vi "MFLIcontrol.vi"(6 "SigIns0 Autorange":bool, 7 "Value":dbl, 8 "error in":errorcluster, 10 "MFLI function":T2, 11 "handle in":T3 {"Handle" format="0x%08x"; "Conn" format="0x%08x"}) -> (0 "error out":errorcluster, 1 "Demod Sample Out 2":T1={"Timestamps (ticks)"=0, "X (Vrms)"=nan, "Y (Vrms)"=nan, "Osc Phase (deg)"=nan, "Freq (Hz)"=nan, "DIO"=0, "AuxIn0 (V)"=nan, "AuxIn1 (V)"=nan, "Trigger"=0}, 2 "Demod Sample Out 3":T1={"Timestamps (ticks)"=0, "X (Vrms)"=nan, "Y (Vrms)"=nan, "Osc Phase (deg)"=nan, "Freq (Hz)"=nan, "DIO"=0, "AuxIn0 (V)"=nan, "AuxIn1 (V)"=nan, "Trigger"=0}, 3 "handle out":T3 {"Handle" format="0x%08x"; "Conn" format="0x%08x"}, 4 "AuxOut0_Ampl":dbl)   [LabVIEW 2021]
uses:
  <instrlib>/Zurich Instruments LabOne/Public/ziTypeHandle.ctl
  MFLIcommand.ctl
  <instrlib>/Zurich Instruments LabOne/Public/Data/ziTypeDemodSampleSingle.ctl
  <instrlib>/Zurich Instruments LabOne/Public/Configure/ziGetValueDemodSampleEx.vi
  <instrlib>/Zurich Instruments LabOne/Public/Configure/ziSetValueDouble.vi
  <instrlib>/Zurich Instruments LabOne/Public/Configure/ziGetValueDouble.vi
  <instrlib>/Zurich Instruments LabOne/Zurich Instruments LabOne.lvlib
panel:
  out "Demod Sample Out 5":T1={"Timestamps (ticks)"=0, "X (Vrms)"=nan, "Y (Vrms)"=nan, "Osc Phase (deg)"=nan, "Freq (Hz)"=nan, "DIO"=0, "AuxIn0 (V)"=nan, "AuxIn1 (V)"=nan, "Trigger"=0}
  out "Demod Sample Out 4":T1={"Timestamps (ticks)"=0, "X (Vrms)"=nan, "Y (Vrms)"=nan, "Osc Phase (deg)"=nan, "Freq (Hz)"=nan, "DIO"=0, "AuxIn0 (V)"=nan, "AuxIn1 (V)"=nan, "Trigger"=0}
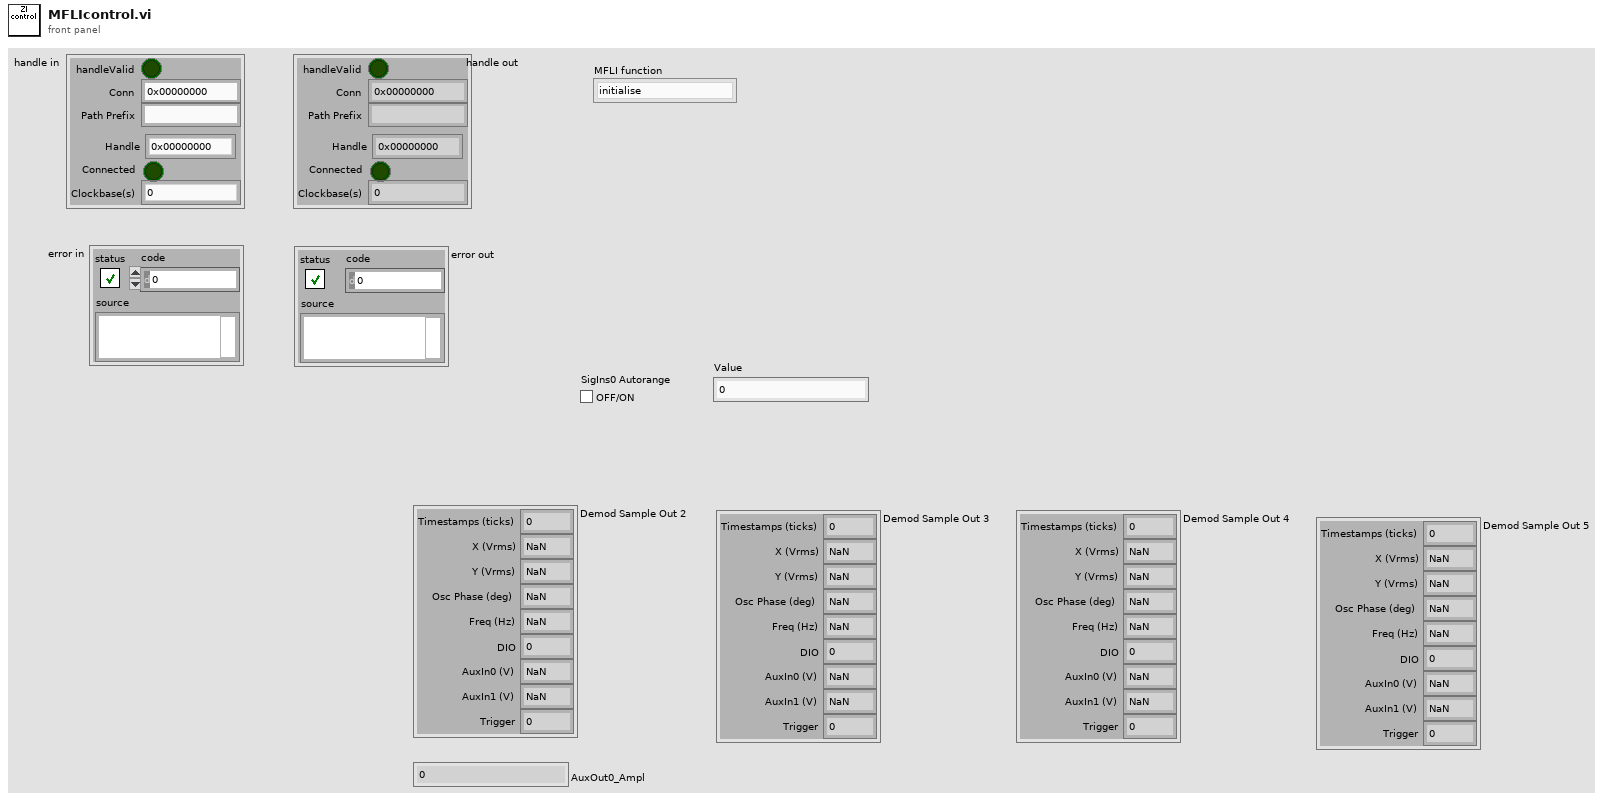
[diagram p1: front panel]
types:
  T1 = typedef "Zurich Instruments LabOne.lvlib/ziTypeDemodSampleSingle.ctl" = cluster{"Timestamps (ticks)":u64, "X (Vrms)":dbl, "Y (Vrms)":dbl, "Osc Phase (deg)":dbl, "Freq (Hz)":dbl, "DIO":u32, "AuxIn0 (V)":dbl, "AuxIn1 (V)":dbl, "Trigger":u32}
  T2 = typedef "MFLIcommand.ctl" = enum16{"initialise", "measure XY on demod0", "measure XY on demod1", "measure XY on demod2", "measure XY on demod3", "Set AuxOut0", "Set AuxOut1", "Set AuxOut2", "Set AuxOut3", "Get AuxOut0", "Set Osc0 Ampl", "Set Osc1 Ampl", "Set Osc0 Freq", "Set Osc1 Freq", "SigIns Autorange", "finalise"}
  T3 = typedef "Zurich Instruments LabOne.lvlib/ziTypeHandle.ctl" = cluster{"handleValid":bool, "Conn":u64, "Path Prefix":string, "Handle":u64, "Connected":bool, "Clockbase(s)":dbl}
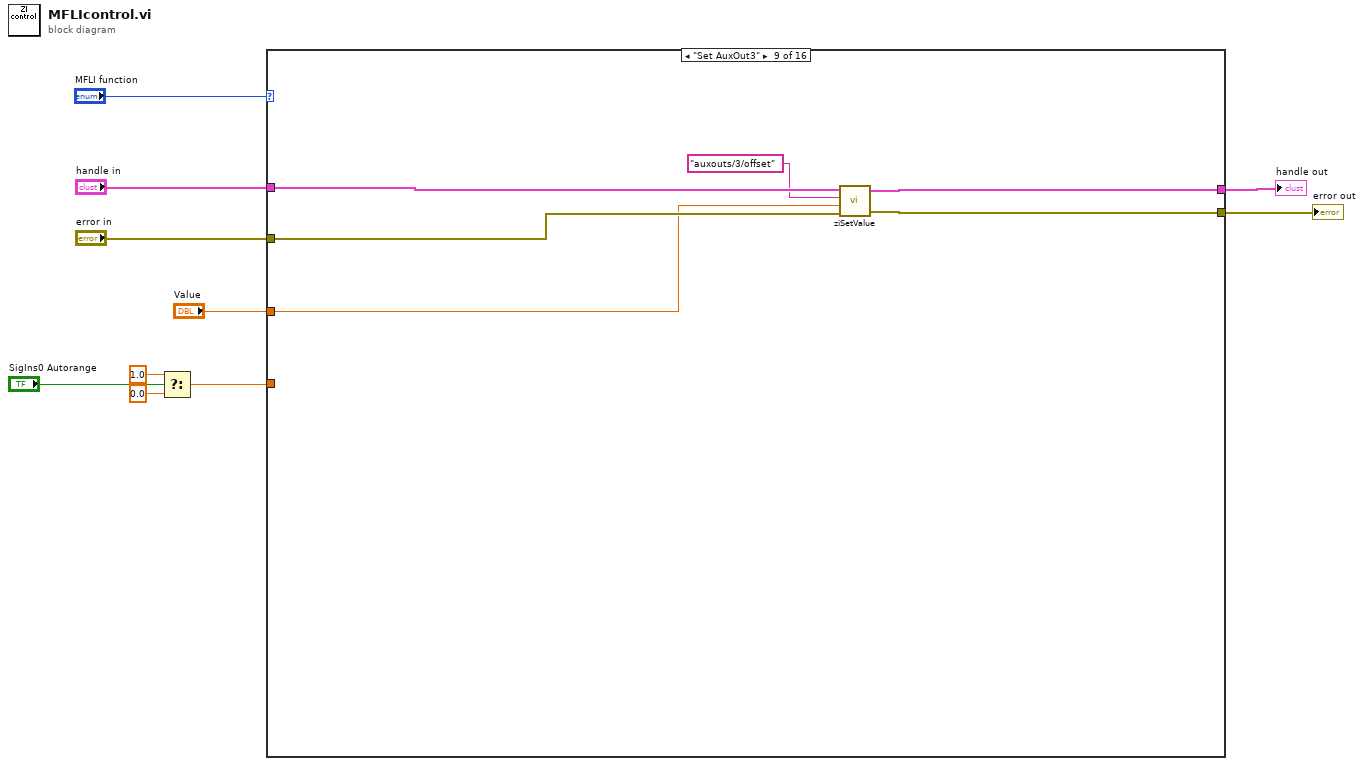
[diagram p0: block diagram]
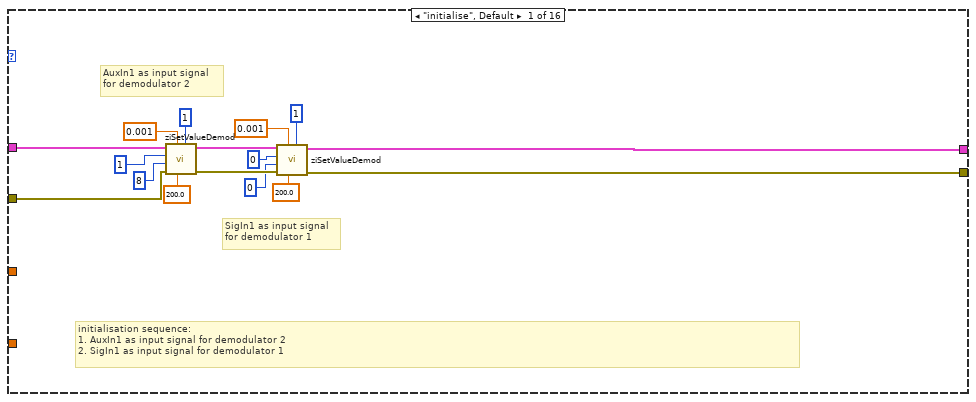
[diagram p2: hidden frame]
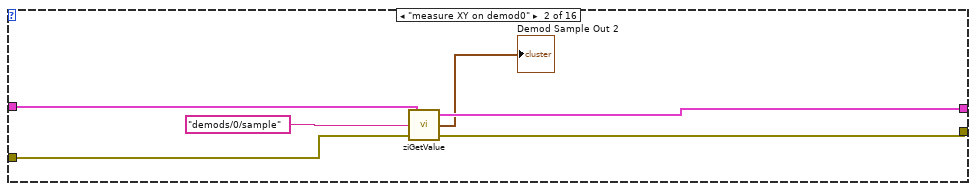
[diagram p3: hidden frame]
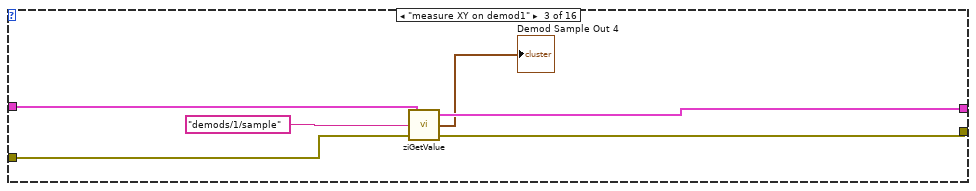
[diagram p4: hidden frame]
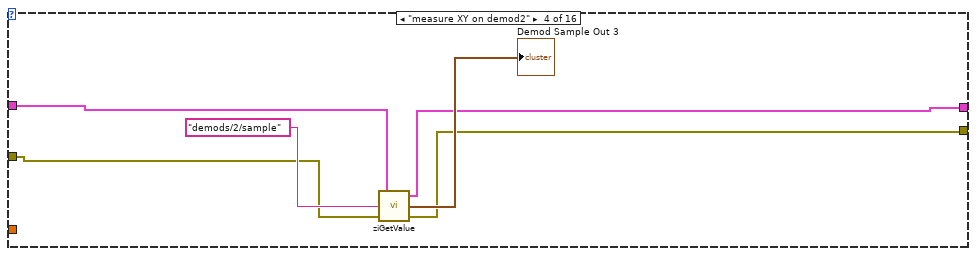
[diagram p5: hidden frame]
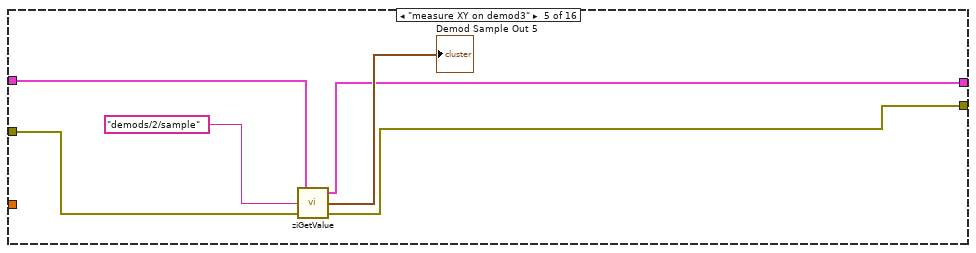
[diagram p6: hidden frame]
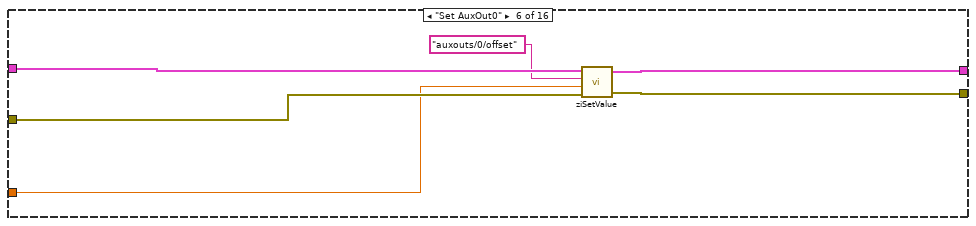
[diagram p7: hidden frame]
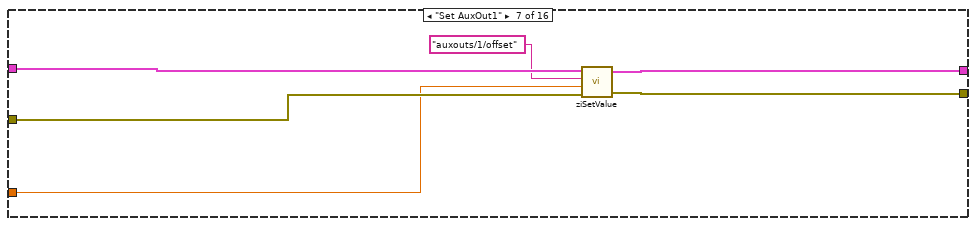
[diagram p8: hidden frame]
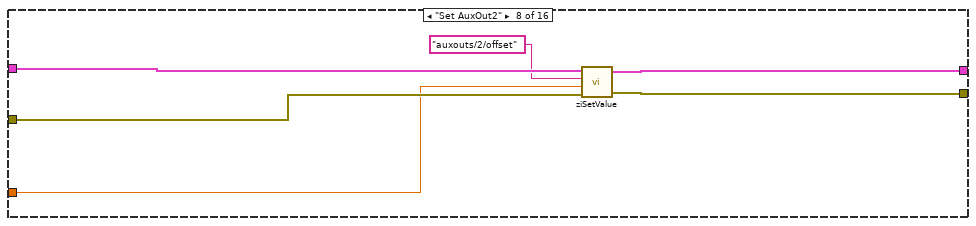
[diagram p9: hidden frame]
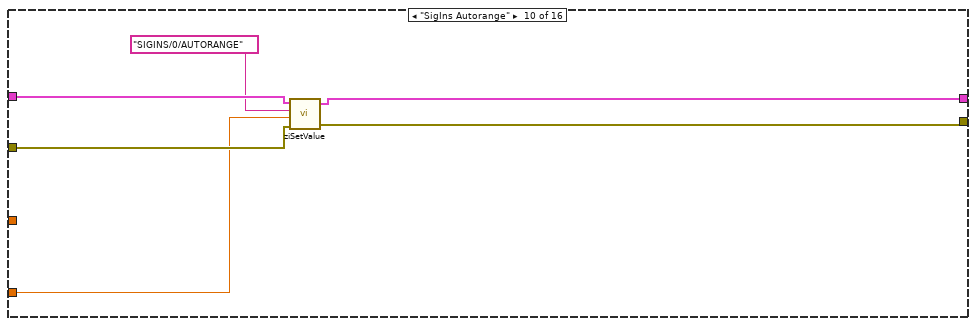
[diagram p10: hidden frame]
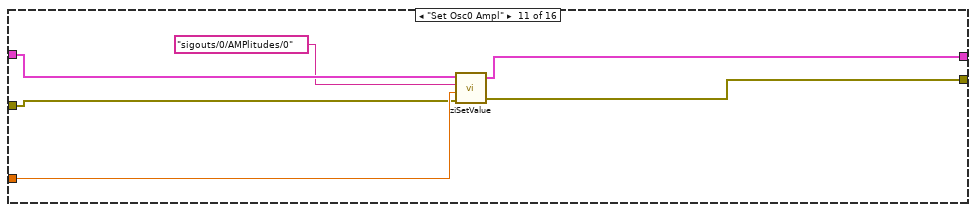
[diagram p11: hidden frame]
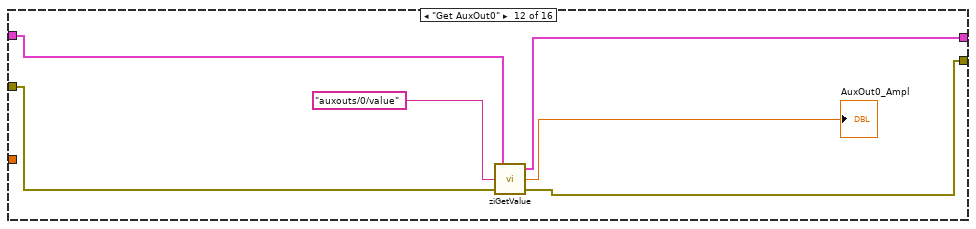
[diagram p12: hidden frame]
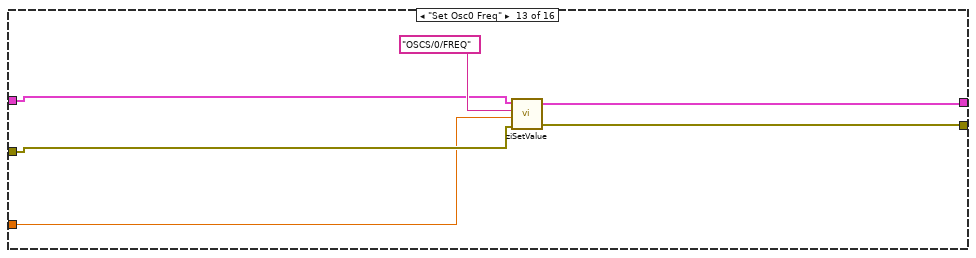
[diagram p13: hidden frame]
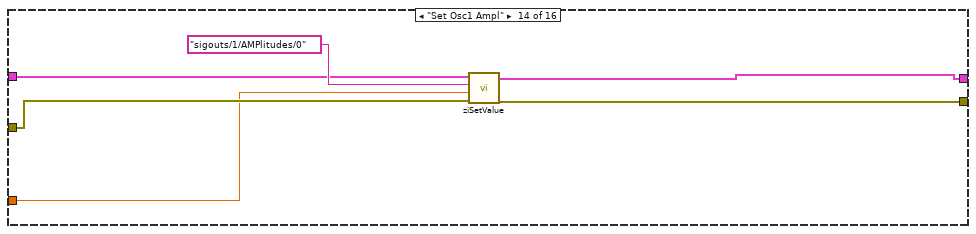
[diagram p14: hidden frame]
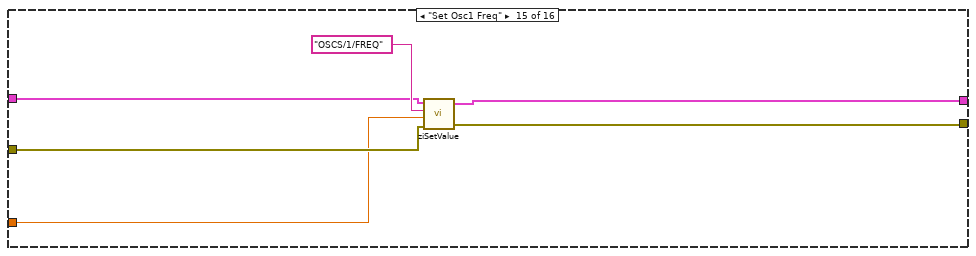
[diagram p15: hidden frame]
diagram:
  n1 = Select(t=1.0, s="SigIns0 Autorange", f=0.0) -> (s? t:f=w1:dbl)
  n2 = case shown="\"Set AuxOut3\"" "MFLI function" {
    tunnel: "handle in" -> [w26 w32 w38 w42 w48 w56 w62 w68 w74 w80 w86 w90 w97 w103 w108 w112]
    tunnel: "error in" -> [w25 w30 w36 w41 w45 w55 w61 w67 w73 w79 w83 w91 w96 w102 w109 w111]
    tunnel: [w24 w29 w35 w40 w47 w54 w60 w66 w72 w78 w82 w88 w95 w99 w106 w112] -> w8
    tunnel: [w23 w28 w34 w39 w46 w53 w59 w65 w71 w77 w81 w89 w94 w100 w105 w111] -> w7
    tunnel: "Value" -> [_ _ _ _ _ w51 w57 w63 w69 _ w84 _ w93 w101 w107 _]
    tunnel: w1 -> [_ _ _ _ _ _ _ _ _ w75 _ _ _ _ _ _]
    frame "initialise", Default {
      # "initialisation sequence:\n1. AuxIn1 as input signal for demodulator 2 \n2. SigIn1 as input signal for demodulator 1"
      # "SigIn1 as input signal \nfor demodulator 1"
      # "AuxIn1 as input signal \nfor demodulator 2"
      n3 = call <instrlib>:"ziSetValueDemod.vi"("Order (2)"=1, "Rate (200Hz)"=200.0, "Time Constant (1ms)"=0.001, "error in"=w25, "Signal Input Select (0)"=8, "Demodulator # (0)"=1, "handle in"=w26) -> ("error out"=w16:errorcluster, "handle out"=w17:T3)  [unwired: 3 in]
      n4 = call <instrlib>:"ziSetValueDemod.vi"("Order (2)"=1, "Rate (200Hz)"=200.0, "Time Constant (1ms)"=0.001, "error in"=w16, "Signal Input Select (0)"=0, "Demodulator # (0)"=0, "handle in"=w17) -> ("error out"=w23:errorcluster, "handle out"=w24:T3)  [unwired: 3 in]
    }
    frame "measure XY on demod0" {
      n5 = call-poly <instrlib>:"ziGetValue.vi"("error in"=w30, "Path"="demods/0/sample", "Handle In"=w32) -> ("error out"=w28:errorcluster, "Demod Sample Out"=→"Demod Sample Out 2":T1, "Handle Out"=w29:T3)
    }
    frame "measure XY on demod1" {
      n6 = call-poly <instrlib>:"ziGetValue.vi"("error in"=w36, "Path"="demods/1/sample", "Handle In"=w38) -> ("error out"=w34:errorcluster, "Demod Sample Out"=→"Demod Sample Out 4":T1, "Handle Out"=w35:T3)
    }
    frame "measure XY on demod2" {
      n7 = call-poly <instrlib>:"ziGetValue.vi"("error in"=w41, "Path"="demods/2/sample", "Handle In"=w42) -> ("error out"=w39:errorcluster, "Demod Sample Out"=→"Demod Sample Out 3":T1, "Handle Out"=w40:T3)
    }
    frame "measure XY on demod3" {
      n8 = call-poly <instrlib>:"ziGetValue.vi"("error in"=w45, "Path"="demods/2/sample", "Handle In"=w48) -> ("error out"=w46:errorcluster, "Demod Sample Out"=→"Demod Sample Out 5":T1, "Handle Out"=w47:T3)
    }
    frame "Set AuxOut0" {
      n9 = call-poly <instrlib>:"ziSetValue.vi"("Error In"=w55, "Value"=w51, "Path"="auxouts/0/offset", "Handle In"=w56) -> ("Error Out"=w53:errorcluster, "Handle Out"=w54:T3)  [unwired: 1 in]
    }
    frame "Set AuxOut1" {
      n10 = call-poly <instrlib>:"ziSetValue.vi"("Error In"=w61, "Value"=w57, "Path"="auxouts/1/offset", "Handle In"=w62) -> ("Error Out"=w59:errorcluster, "Handle Out"=w60:T3)  [unwired: 1 in]
    }
    frame "Set AuxOut2" {
      n11 = call-poly <instrlib>:"ziSetValue.vi"("Error In"=w67, "Value"=w63, "Path"="auxouts/2/offset", "Handle In"=w68) -> ("Error Out"=w65:errorcluster, "Handle Out"=w66:T3)  [unwired: 1 in]
    }
    frame "Set AuxOut3" {
      n12 = call-poly <instrlib>:"ziSetValue.vi"("Error In"=w73, "Value"=w69, "Path"="auxouts/3/offset", "Handle In"=w74) -> ("Error Out"=w71:errorcluster, "Handle Out"=w72:T3)  [unwired: 1 in]
    }
    frame "SigIns Autorange" {
      n13 = call-poly <instrlib>:"ziSetValue.vi"("Error In"=w79, "Value"=w75, "Path"="SIGINS/0/AUTORANGE", "Handle In"=w80) -> ("Error Out"=w77:errorcluster, "Handle Out"=w78:T3)  [unwired: 1 in]
    }
    frame "Set Osc0 Ampl" {
      n14 = call-poly <instrlib>:"ziSetValue.vi"("Error In"=w83, "Value"=w84, "Path"="sigouts/0/AMPlitudes/0", "Handle In"=w86) -> ("Error Out"=w81:errorcluster, "Handle Out"=w82:T3)  [unwired: 1 in]
    }
    frame "Get AuxOut0" {
      n15 = call-poly <instrlib>:"ziGetValue.vi"("error in"=w91, "Path"="auxouts/0/value", "Handle in"=w90) -> ("error out"=w89:errorcluster, "Value"=→"AuxOut0_Ampl":dbl, "Handle out"=w88:T3)
    }
    frame "Set Osc0 Freq" {
      n16 = call-poly <instrlib>:"ziSetValue.vi"("Error In"=w96, "Value"=w93, "Path"="OSCS/0/FREQ", "Handle In"=w97) -> ("Error Out"=w94:errorcluster, "Handle Out"=w95:T3)  [unwired: 1 in]
    }
    frame "Set Osc1 Ampl" {
      n17 = call-poly <instrlib>:"ziSetValue.vi"("Error In"=w102, "Value"=w101, "Path"="sigouts/1/AMPlitudes/0", "Handle In"=w103) -> ("Error Out"=w100:errorcluster, "Handle Out"=w99:T3)  [unwired: 1 in]
    }
    frame "Set Osc1 Freq" {
      n18 = call-poly <instrlib>:"ziSetValue.vi"("Error In"=w109, "Value"=w107, "Path"="OSCS/1/FREQ", "Handle In"=w108) -> ("Error Out"=w105:errorcluster, "Handle Out"=w106:T3)  [unwired: 1 in]
    }
    frame "finalise" {
    }
  }
  "handle out" <- w8
  "error out" <- w7
